vi "GE 5565PIORC.DMA.Block.vi"(11 "count (1000)":u32=1000) -> (0 "error out":errorcluster, 3 "pass?":bool)   [LabVIEW 2020]
uses:
  Source/GE 5565PIORC.lvclass/GE 5565PIORC.ctl
  Source/Methods/GE 5565PIORC.DMA.Block.Write (DBL).vi
  Source/Methods/GE 5565PIORC.DMA.Create Transfer (Block).vi
  Source/Methods/GE 5565PIORC.DMA.Block.Read (DBL).vi
  Source/Properties/Registers/GE 5565PIORC.Registers.DMACSR0.Channel 0 Enable.Set.vi
  Source/Properties/GE 5565PIORC.Read VISA MEMACC.vi
  Source/Methods/GE 5565PIORC.DMA.Create Transfer (Scatter-Gather).vi
  Source/Methods/GE 5565PIORC.DMA.Configure.vi
  Source/Methods/GE 5565PIORC.PXI Interrupts.Discard Events.vi
  Source/Methods/GE 5565PIORC.DMA.Start.vi
  Source/Methods/GE 5565PIORC.DMA.Wait for Done.vi
  Source/Properties/Registers/GE 5565PIORC.Registers.Local Configuration.Read.vi
  Source/Properties/Registers/GE 5565PIORC.Registers.Local Configuration.Read (U8).vi
  Source/Properties/Registers/GE 5565PIORC.Registers.Local Configuration.Write.vi
  Source/Properties/Registers/GE 5565PIORC.Registers.Local Configuration.Write (U8).vi
  Source/Methods/GE 5565PIORC.Bit Manipulation.Set Bit.vi
  Source/Methods/GE 5565PIORC.Bit Manipulation.Set Bit (U8).vi
  Source/Methods/GE 5565PIORC.DMA.Size.vi
  Source/Properties/Registers/GE 5565PIORC.Registers.DMADPR0.Direction of Transfer.Set.vi
  Source/Properties/Registers/GE 5565PIORC.Registers.DMASIZ0.DMA Transfer Size.Set.vi
  Source/Properties/Registers/GE 5565PIORC.Registers.DMALADR0.Local Address Register.Set.vi
  Source/Properties/Registers/GE 5565PIORC.Registers.DMAMODE0.Scatter-Gather Mode.Set.vi
  Source/Properties/Registers/GE 5565PIORC.Registers.DMAPADR0.PCI Address Register.Set.vi
  Source/Methods/GE 5565PIORC.DMA.Scatter-Gather.Link Block Descriptors.vi
  Source/Methods/GE 5565PIORC.DMA.Scatter-Gather.Commit Linked Block Descriptors.vi
  Source/Properties/Registers/GE 5565PIORC.Registers.DMADPR0.Channel 0 First Descriptor Address.Set.vi
  Source/Methods/GE 5565PIORC.DMA.Get Transfer Components.vi
  Source/Methods/GE 5565PIORC.DMA.Get Transfer Components (Scatter-Gather).vi
  <vilib>/Utility/error.llb/Clear Errors.vi
  Source/Properties/Registers/GE 5565PIORC.Registers.DMACSR0.Channel 0 Start.Set.vi
  Source/Properties/Registers/GE 5565PIORC.Registers.DMACSR0.Channel 0 Clear Interrupt.Set.vi
  Source/Methods/GE 5565PIORC.DMA.Poll for Done Signal.vi
  Source/Methods/GE 5565PIORC.PXI Interrupts.Wait for Event.vi
  Source/Methods/GE 5565PIORC.Registers.Read.vi
  Source/Methods/GE 5565PIORC.Registers.Read (U8).vi
  Source/Methods/GE 5565PIORC.Registers.Write.vi
  Source/Methods/GE 5565PIORC.Registers.Write (U8).vi
  Source/Properties/Registers/GE 5565PIORC.Registers.Local Configuration.Read (U32).vi
  Source/Properties/Registers/GE 5565PIORC.Registers.Local Configuration.Write (U32).vi
  Source/Methods/GE 5565PIORC.Bit Manipulation.Set Bit (U32).vi
  Source/Methods/GE 5565PIORC.DMA.Scatter-Gather.Set Descriptor Params.vi
  Source/Methods/GE 5565PIORC.DMA.Is Done.vi
  Source/Methods/GE 5565PIORC.Registers.Read (U32).vi
  Source/Methods/GE 5565PIORC.Registers.Write (U32).vi
  Source/Properties/Registers/GE 5565PIORC.Registers.DMACSR0.Channel 0 Inactive.Get.vi
  Source/Methods/GE 5565PIORC.Bit Manipulation.Get Bit.vi
  Source/Methods/GE 5565PIORC.Bit Manipulation.Get Bit (U8).vi
  Source/Methods/GE 5565PIORC.Round Up to Nearest 8.vi
  Source/Methods/GE 5565PIORC.Round Up to Nearest 16.vi
  Source/GE 5565PIORC.lvclass
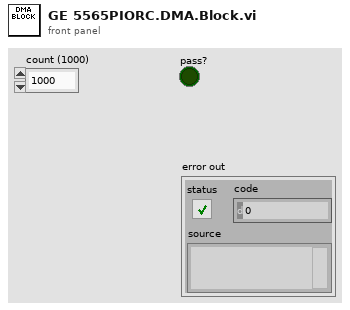
[diagram p1: front panel]
types:
  T1 = typedef "GE 5565PIORC.lvclass/GE 5565PIORC.Typedef.DMA Block Descriptor.ctl" = cluster{"descriptor ptr (VISA)":u32, "descriptor ptr (RFM)":u32, "descriptor size":u32, "descriptor params":T2}
  T2 = typedef "GE 5565PIORC.lvclass/GE 5565PIORC.Typedef.DMA Block Descriptor Params.ctl" = cluster{"data ptr (lower)":u32, "data ptr (upper)":u32, "data size":u32, "next descriptor ptr":u32}
  T3 = typedef "GE 5565PIORC.lvclass/GE 5565PIORC.Typedef.DMA Transfer Spec.ctl" = cluster{"RFM offset":u32, "Block Descriptors":T1[]}
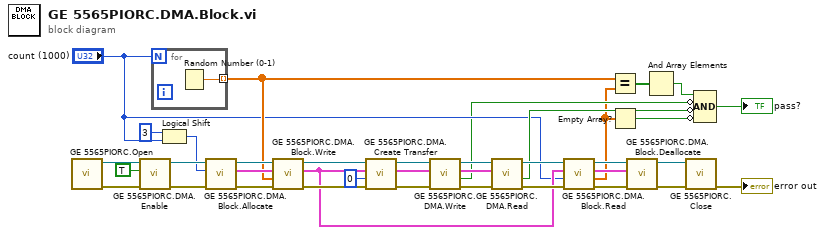
[diagram p0: block diagram]
diagram:
  n1 = call "GE 5565PIORC.Open.vi"() -> ("error out"=w1:errorcluster, "GE 5565PIORC"=w2:refnum<class "GE 5565PIORC.lvclass">)  [unwired: 10 in]
  n2 = call "GE 5565PIORC.DMA.Enable.vi"("error in (no error)"=w1, "enable (T)"=TRUE ("Enable DMA"), "GE 5565PIORC in"=w2) -> ("error out"=w34:errorcluster, "GE 5565PIORC out"=w35:refnum<class "GE 5565PIORC.lvclass">)  [unwired: 7 in]
  n3 = for {
    N: "count (1000)" -> [_]
    tunnel: [w38] -> w19 mode=indexing
    n4 = Random Number (0-1)() -> (number: 0 to 1=w38:dbl)
  }
  n5 = Logical Shift(y=i16 3, x="count (1000)") -> (x << y=w29:u32)
  n6 = call "GE 5565PIORC.DMA.Block.Allocate.vi"("error in (no error)"=w34, "size in bytes"=w29, "GE 5565PIORC in"=w35) -> ("error out"=w31:errorcluster, "Block Descriptor"=w30:T1, "GE 5565PIORC out"=w32:refnum<class "GE 5565PIORC.lvclass">)  [unwired: 6 in]
  n7 = call-poly "GE 5565PIORC.DMA.Block.Write.vi"("error in (no error)"=w31, "data"=w19, "Block Descriptor in"=w30, "GE 5565PIORC in"=w32) -> ("error out"=w26:errorcluster, "Block Descriptor out"=w23:T1, "GE 5565PIORC out"=w27:refnum<class "GE 5565PIORC.lvclass">)  [unwired: 4 in, 1 out]
  n8 = call-poly "GE 5565PIORC.DMA.Create Transfer.vi"("error in (no error)"=w26, "RFM offset"=u32 0, "Block Descriptor"=w23, "GE 5565PIORC in"=w27) -> ("error out"=w10:errorcluster, "DMA Transfer Spec"=w9:T3, "GE 5565PIORC out"=w11:refnum<class "GE 5565PIORC.lvclass">)  [unwired: 4 in, 1 out]
  n9 = call "GE 5565PIORC.DMA.Write.vi"("error in (no error)"=w10, "DMA Transfer Spec"=w9, "GE 5565PIORC in"=w11) -> ("error out"=w6:errorcluster, "timed out?"=w5:bool, "DMA Transfer Spec dup"=w8:T3, "GE 5565PIORC out"=w7:refnum<class "GE 5565PIORC.lvclass">)  [unwired: 5 in]
  n10 = call "GE 5565PIORC.DMA.Read.vi"("error in (no error)"=w6, "DMA Transfer Spec"=w8, "GE 5565PIORC in"=w7) -> ("error out"=w24:errorcluster, "timed out?"=w18:bool, "GE 5565PIORC out"=w25:refnum<class "GE 5565PIORC.lvclass">)  [unwired: 5 in, 1 out]
  n11 = call-poly "GE 5565PIORC.DMA.Block.Read.vi"("error in (no error)"=w24, "count"="count (1000)", "Block Descriptor in"=w23, "GE 5565PIORC in"=w25) -> ("error out"=w20:errorcluster, "data out"=w4:dbl[], "Block Descriptor out"=w21:T1, "GE 5565PIORC out"=w22:refnum<class "GE 5565PIORC.lvclass">)  [unwired: 4 in]
  n12 = Equal?(x=w19, y=w4) -> (x = y?=w17:bool[])
  n13 = Empty Array?(array=w4) -> (empty?=w3:bool)
  n14 = call "GE 5565PIORC.DMA.Block.Deallocate.vi"("error in (no error)"=w20, "Block Descriptor"=w21, "GE 5565PIORC in"=w22) -> ("error out"=w14:errorcluster, "GE 5565PIORC out"=w15:refnum<class "GE 5565PIORC.lvclass">)  [unwired: 7 in]
  n15 = And Array Elements(Boolean array=w17) -> (logical AND=w16:bool)
  n16 = call "GE 5565PIORC.Close.vi"("error in (no error)"=w14, "GE 5565PIORC"=w15) -> ("error out"=→"error out":errorcluster)  [unwired: 9 in]
  n17 = Compound Arithmetic op=AND(w16, invert w5, invert w18, invert w3) -> (→"pass?":bool)
